vi "Open TDMS.vi"(7 "Operation (0:open)":T1(ring), 8 "error in (no error)":errorcluster, 9 "Group":string, 10 "File Path":path, 11 "Honeywell Compass HMC6343":refnum<class "Honeywell Compass HMC6343.lvclass">) -> (0 "error out":errorcluster, 3 "Honeywell Compass HMC6343 out":refnum<class "Honeywell Compass HMC6343.lvclass">)   [LabVIEW 2019, in "Honeywell Compass HMC6343.lvclass"]
doc: "Opens a TDMS file."
uses:
  Honeywell Compass HMC6343.lvclass
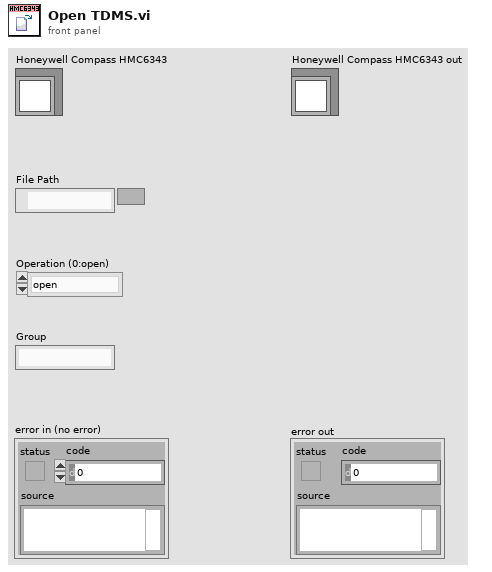
[diagram p1: front panel]
types:
  T1 = enum16{"open", "open or create", "create or replace", "create", "open (read-only)"}
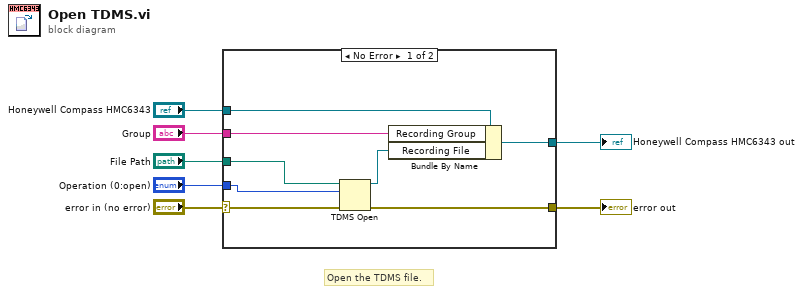
[diagram p0: block diagram]
diagram:
  # "Open the TDMS file."
  n1 = case shown="No Error" "error in (no error)" {
    selector: "error in (no error)" -> [w15 w17]
    tunnel: "File Path" -> [w14 _]
    tunnel: "Operation (0:open)" -> [w13 _]
    tunnel: "Honeywell Compass HMC6343" -> [w12 w16]
    tunnel: [w11 w17] -> w3
    tunnel: [w10 w16] -> w2
    tunnel: "Group" -> [w8 _]
    frame No Error {
      n2 = TDMS Open(8:w15, 10:w13, 11:w14) -> (0:w11:errorcluster, 3:w9:refnum<k34>)  [unwired: 4 in]
      n3 = Bundle By Name(cluster=w12, "Recording Group"=w8, "Recording File"=w9) -> (w10:refnum<class "Honeywell Compass HMC6343.lvclass">)
    }
    frame Error {
    }
  }
  "error out" <- w3
  "Honeywell Compass HMC6343 out" <- w2
